vi "_processKafkaMessage - Copy.vi"(8 "error in (no error)":errorcluster, 11 "Kafka Events":T1[](array[typedef])) -> (0 "error out":errorcluster, 3 "Array":cluster{"Key":string, "value":T1[]}[](array[cluster]))   [LabVIEW 2019]
uses:
  KafkaLVLib/API/KafkaConsumerEvent.ctl
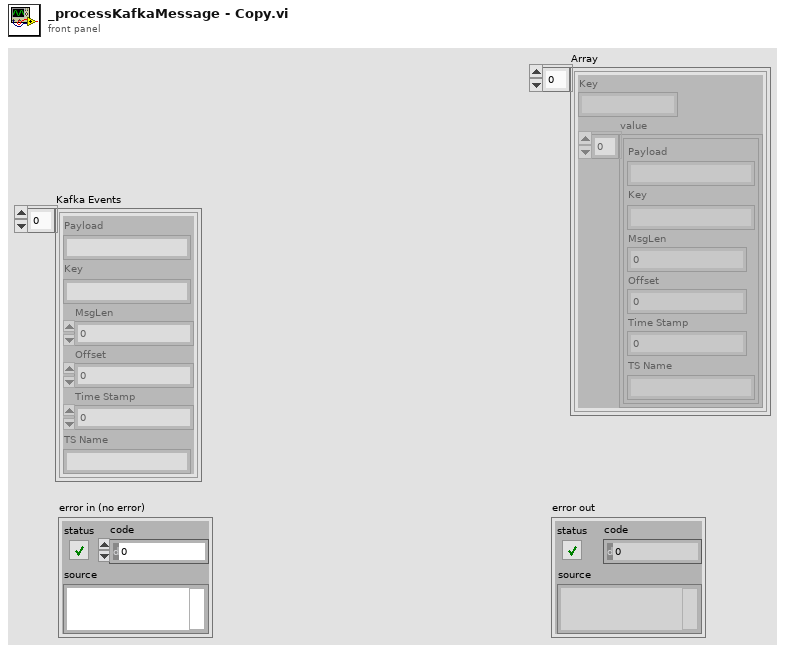
[diagram p1: front panel]
types:
  T1 = typedef "KafkaConsumerEvent.ctl" = cluster{"Payload":string, "Key":string, "MsgLen":u64, "Offset":i64, "Time Stamp":i64, "TS Name":string}
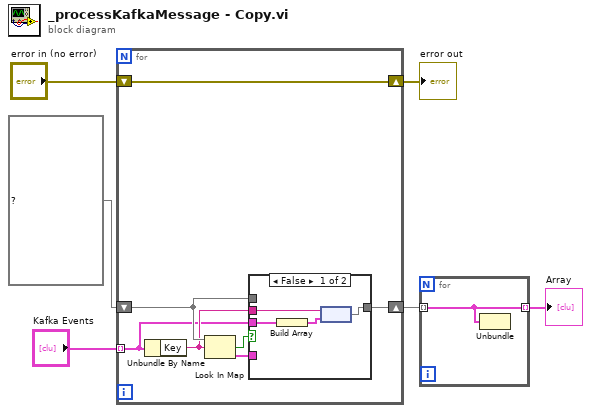
[diagram p0: block diagram]
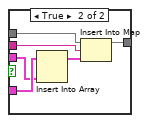
[diagram p2: hidden frame]
diagram:
  n1 = for {
    shift-right: [w7] -> w5
    shift-left: "error in (no error)" -> [w7]
    tunnel: "Kafka Events" -> [w8] mode=indexing
    shift-right: [w11] -> w3
    shift-left: map{string, T1[]} {} ("map") -> [w12]
    n2 = Unbundle By Name(w8) -> ("Key"=w10:string)
    n3 = Look In Map(map=w12, key=w10) -> (key not found?=w13:bool, value=w9:T1[])  [unwired: 1 in]
    n4 = case shown="False" w13 {
      tunnel: w12 -> [_ w23]
      tunnel: [w14 w22] -> w11
      tunnel: w10 -> [w17 w21]
      tunnel: w9 -> [_ w20]
      tunnel: w8 -> [w16 w19]
      frame False {
        n5 = Build Array(w16) -> (w15:T1[])
        n6 = node(w17, w15) -> (w14:map{string, T1[]})
      }
      frame True {
        n7 = Insert Into Array(array=w20, new element=w19) -> (w18:T1[])  [unwired: 1 in]
        n8 = Insert Into Map(map in=w23, key=w21, value=w18) -> (map out=w22:map{string, T1[]})  [unwired: 2 out]
      }
    }
  }
  "error out" <- w5
  n9 = for {
    tunnel: [w24] -> w2 mode=indexing
    tunnel: w3 -> [w24] mode=indexing
    n10 = Unbundle(w24) -> ()  [unwired: 2 out]
  }
  "Array" <- w2
